vi "sv_UFF58 Set Record Fields (Time).vi"(0 "ID lines (1-3)":T4, 1 "waveform":waveform(dbl)={"t0"=timestamp(0 s since 1904-01-01), "dt"=0.0, "Y"=[]}, 2 "function type":T1=enum."time response" caption="function data type", 5 "error in (no error)":errorcluster) -> (7 "DOF identification (record 6)":T5 {"reference direction" items=["-Z Rotation"=-6, "-Y Rotation"=-5, "-X Rotation"=-4, "-Z Translation"=-3, "-Y Translation"=-2, "-X Translation"=-1, "Scalar"=0, "+X Translation"=1, "+Y Translation"=2, "+Z Translation"=3, "+X Rotation"=4, "+Y Rotation"=5, "+Z Rotation"=6]; "response direction" items=["-Z Rotation"=-6, "-Y Rotation"=-5, "-X Rotation"=-4, "-Z Translation"=-3, "-Y Translation"=-2, "-X Translation"=-1, "Scalar"=0, "+X Translation"=1, "+Y Translation"=2, "+Z Translation"=3, "+X Rotation"=4, "+Y Rotation"=5, "+Z Rotation"=6]}, 9 "abscissa data characteristics (record 8)":T2 {"specific data type" items=["unknown"=0, "general"=1, "stress"=2, "strain"=3, "temperature"=5, "heat flux"=6, "displacement"=8, "reaction force"=9, "velocity"=11, "acceleration"=12, "excitation force"=13, "pressure"=15, "mass"=16, "time"=17, "frequency"=18, "rpm"=19, "order"=20, "sound pressure"=21, "sound intensity"=22, "sound power"=23]}, 11 "ordinate numerator data characteristics (record 9)":T2 {"specific data type" items=["unknown"=0, "general"=1, "stress"=2, "strain"=3, "temperature"=5, "heat flux"=6, "displacement"=8, "reaction force"=9, "velocity"=11, "acceleration"=12, "excitation force"=13, "pressure"=15, "mass"=16, "time"=17, "frequency"=18, "rpm"=19, "order"=20, "sound pressure"=21, "sound intensity"=22, "sound power"=23]}, 12 "ID lines (1-3) out":T4, 14 "dup waveform":waveform(dbl), 19 "error out":errorcluster)   [LabVIEW 2017, in "SoundVib_UFF58.lvlib"]
doc: "This VI sets the following record values:\nRecords (1-3) (name): <B>ID lines (1-3) out</B>\nRecord 6 (function type): <B>DOF identification (record 6)</B>\nRecord 8 (specific data type, axis label, unit label): <B>abscissa data characteristics (record 8)</B>\nRecord 9 (specific data type, axis label, unit label): <B>ordinate numerator data characteristics (record 9)</B>"
uses:
  <vilib>/addons/Sound and Vibration/svt_UFF58/SoundVib_UFF58.lvlib
  <vilib>/addons/Sound and Vibration/svt_UFF58/subVIs/sv_UFF58 Axis Characteristics.ctl
  <vilib>/addons/Sound and Vibration/svt_UFF58/subVIs/sv_UFF58 Specific Datatype.ctl
  <vilib>/addons/Sound and Vibration/svt_UFF58/subVIs/sv_UFF58 DOF.ctl
  <vilib>/addons/Sound and Vibration/svt_UFF58/subVIs/sv_FunctionType.ctl
  <vilib>/addons/Sound and Vibration/svt_UFF58/subVIs/sv_UFF58 Response Direction.ctl
  <vilib>/addons/Sound and Vibration/svt_UFF58/subVIs/sv_IDLines123.ctl
  <vilib>/addons/_NISVFA/_Shared subVIs/Common/svc_Engineering Units to Unit Label.vi
  <vilib>/addons/_NISVFA/_Shared subVIs/Common/svc_Unit Label to Engineering Units.vi
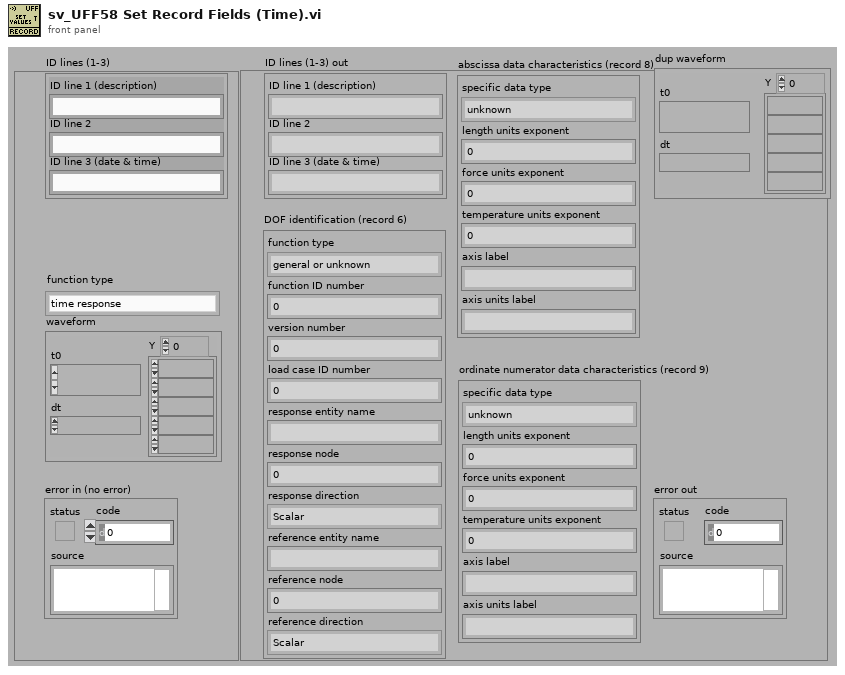
[diagram p1: front panel]
types:
  T1 = typedef "SoundVib_UFF58.lvlib/sv_FunctionType.ctl" = enum16{"general or unknown", "time response", "auto spectrum", "cross spectrum", "frequency response function", "transmissibility", "coherence", "auto correlation", "cross correlation", "power spectral density (PSD)", "energy spectral density (ESD)", "probability density function", "spectrum", "cumulative frequency distribution", "peaks valley", "stress/cycles", "strain/cycles", "orbit", "mode indicator function", "force pattern", "partial power", "partial coherence", "eigenvalue", "eigenvector", "shock response spectrum", "finite impulse response filter", "multiple coherence", "order function", "phase compensation"}
  T2 = typedef "SoundVib_UFF58.lvlib/sv_UFF58 Axis Characteristics.ctl" = cluster{"specific data type":T3, "length units exponent":i32, "force units exponent":i32, "temperature units exponent":i32, "axis label":string, "axis units label":string}
  T3 = typedef "SoundVib_UFF58.lvlib/sv_UFF58 Specific Datatype.ctl" = u16
  T4 = typedef "SoundVib_UFF58.lvlib/sv_IDLines123.ctl" = cluster{"ID line 1 (description)":string, "ID line 2":string, "ID line 3 (date & time)":string}
  T5 = typedef "SoundVib_UFF58.lvlib/sv_UFF58 DOF.ctl" = cluster{"function type":T1, "function ID number":i32, "version number":i32, "load case ID number":i32, "response entity name":string, "response node":i32, "response direction":T6, "reference entity name":string, "reference node":i32, "reference direction":T6}
  T6 = typedef "SoundVib_UFF58.lvlib/sv_UFF58 Response Direction.ctl" = i32
  T7 = typedef "svc_Channel Info.ctl" = cluster{"sensor sensitivity":dbl, "engineering units":T8, "dB reference":dbl, "custom label":string, "weighting filter":T9, "pregain":dbl}
  T8 = typedef "svc_Engineering Units Text Ring.ctl" = u16
  T9 = typedef "svc_Weighting Filter Text Ring.ctl" = u16
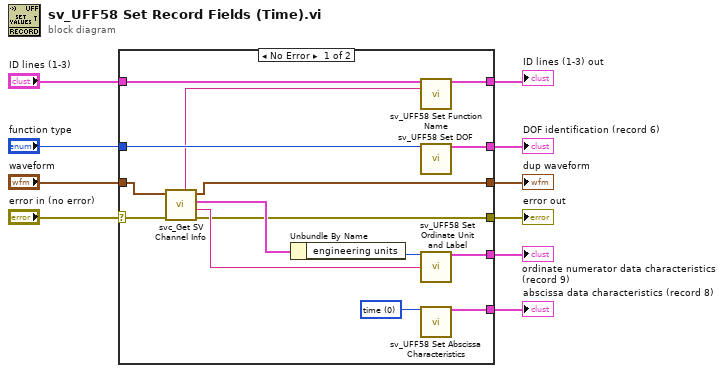
[diagram p0: block diagram]
diagram:
  n1 = case shown="No Error" "error in (no error)" {
    selector: "error in (no error)" -> [w14 w28]
    tunnel: [w25 _] -> w10
    tunnel: [w24 _] -> w9
    tunnel: [w23 w26] -> w8
    tunnel: "ID lines (1-3)" -> [w22 w26]
    tunnel: [w21 _] -> w6
    tunnel: "function type" -> [w20 _]
    tunnel: "waveform" -> [w15 w27]
    tunnel: [w11 w28] -> w3
    tunnel: [w18 w27] -> w1
    frame No Error {
      w17 = u16 0 items=["time"=0, "frequency"=1, "quefrency"=2, "revolutions"=3, "order"=4, "rpm"=11, "rad/s"=21, "index"=65535] ("x-axis units")
      n2 = call <vilib>:"svc_Get SV Channel Info.vi"("error in (no error)"=w14, "scaled signal [EU]"=w15) -> ("error out"=w11:errorcluster, "unit label"=w13:string, "channel info"=w12:T7, "dup scaled signal [EU]"=w18:waveform(dbl), "channel name"=w16:string)  [unwired: 4 in, 1 out]
      n3 = Unbundle By Name(w12) -> ("engineering units"=w19:T8)
      n4 = call <vilib>:"sv_UFF58 Set Function Name.vi"("ID lines (1-3) in"=w22, "channel name"=w16) -> ("ID lines (1-3) out"=w23:T4)  [unwired: 12 in, 1 out]
      n5 = call <vilib>:"sv_UFF58 Set DOF.vi"("function type"=w20) -> ("DOF identification (record 6)"=w24:T5)  [unwired: 14 in]
      n6 = call <vilib>:"sv_UFF58 Set Ordinate Unit and Label.vi"("engineering units"=w19, "unit label"=w13) -> ("ordinate data characteristics (record 9 or 10)"=w21:T2)  [unwired: 13 in]
      n7 = call <vilib>:"sv_UFF58 Set Abscissa Characteristics.vi"("x-axis units"=w17) -> ("abscissa data characteristics (record 8)"=w25:T2)  [unwired: 14 in]
    }
    frame Error {
    }
  }
  "abscissa data characteristics (record 8)" <- w10
  "DOF identification (record 6)" <- w9
  "ID lines (1-3) out" <- w8
  "ordinate numerator data characteristics (record 9)" <- w6
  "error out" <- w3
  "dup waveform" <- w1
